vi "Create Hysteresis Results Summary Table.vi"(8 "error in (no error)":errorcluster, 11 "Hysteresis Results":T1[](array[typedef]) {"Hysteresis Percent FS" format="%#_3g"}) -> (0 "error out":errorcluster, 3 "Hysteresis Table":string[][](array[string]))   [LabVIEW 2026, in "Analysis.lvlib"]
uses:
  Analysis.lvlib
  Hysteresis Result.ctl
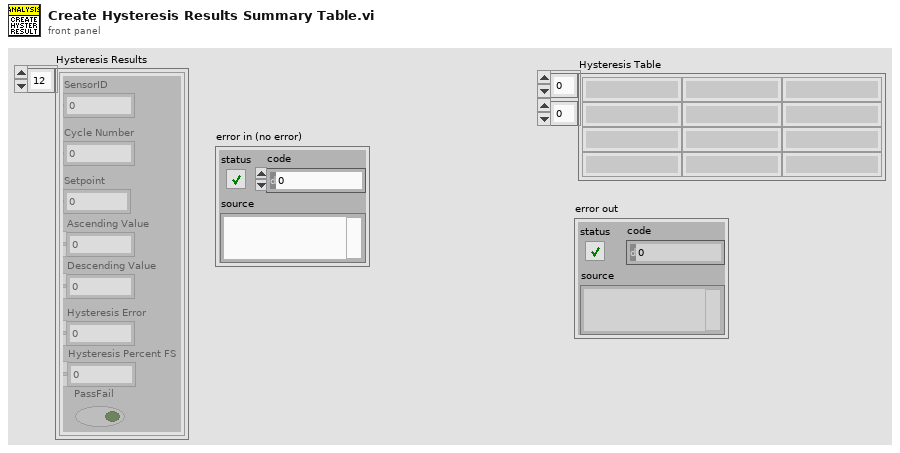
[diagram p1: front panel]
types:
  T1 = typedef "Analysis.lvlib/Hysteresis Result.ctl" = cluster{"Setpoint":dbl, "Ascending Value":dbl, "Cycle Number":i32, "SensorID":i32, "Descending Value":dbl, "Hysteresis Error":dbl, "Hysteresis Percent FS":dbl, "PassFail":bool}
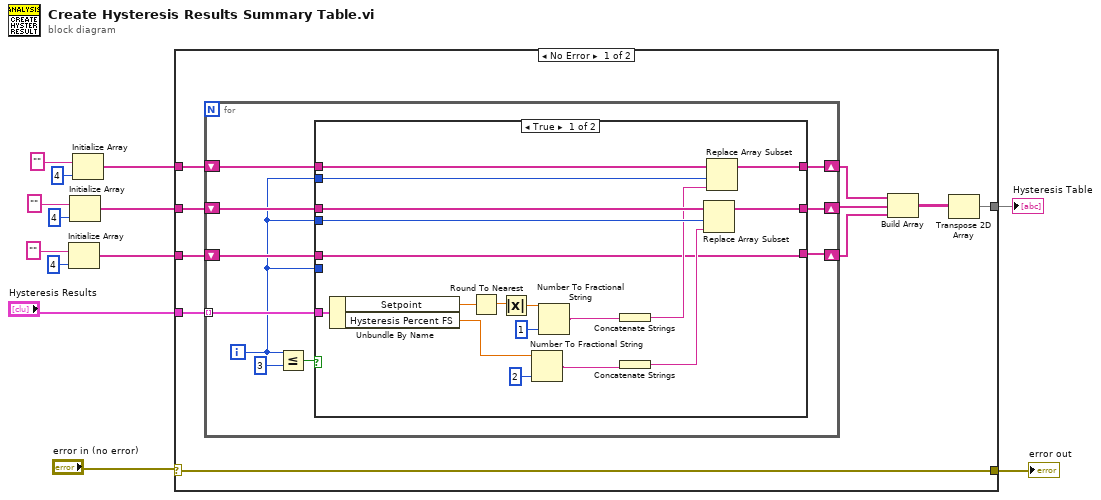
[diagram p0: block diagram]
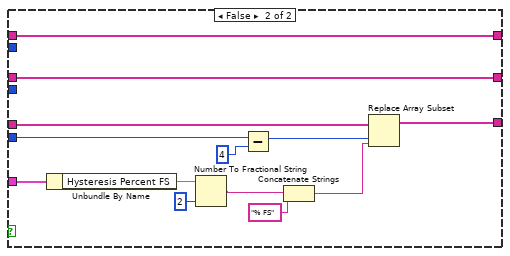
[diagram p2: hidden frame]
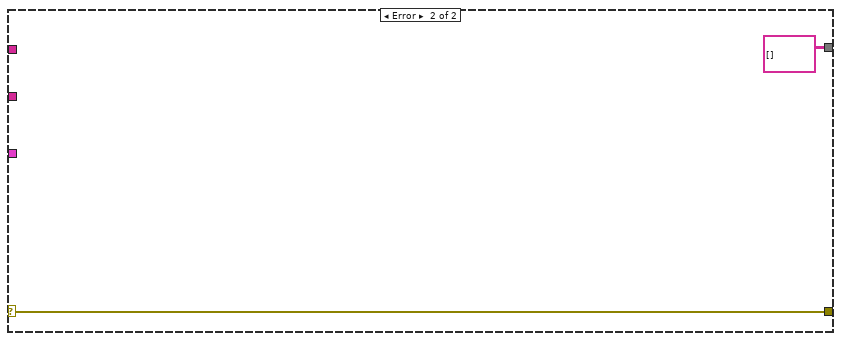
[diagram p3: hidden frame]
diagram:
  n1 = Initialize Array("" ("element"), 4 ("dimension size")) -> (w5:string[])
  n2 = Initialize Array("" ("element"), 4 ("dimension size")) -> (w8:string[])
  n3 = Initialize Array("" ("element"), 4 ("dimension size")) -> (w11:string[])
  n4 = case shown="No Error" "error in (no error)" {
    selector: "error in (no error)" -> [w14 w66]
    tunnel: w11 -> [w23 _]
    tunnel: w8 -> [w22 _]
    tunnel: w5 -> [w21 _]
    tunnel: "Hysteresis Results" -> [w17 _]
    tunnel: [w15 string[][] []] -> w3
    tunnel: [w14 w66] -> w1
    frame No Error {
      n5 = for {
        tunnel: w17 -> [w33] mode=indexing
        shift-right: [w27] -> w20
        shift-left: w23 -> [w30]
        shift-right: [w28] -> w19
        shift-left: w22 -> [w29]
        shift-right: [w24] -> w18
        shift-left: w21 -> [w26]
        i -> [w25]
        n6 = Less Or Equal?(x=w25, y=3) -> (x <= y?=w31:bool)
        n7 = case shown="True" w31 {
          tunnel: w33 -> [w51 w64]
          tunnel: w30 -> [w42 w59]
          tunnel: w29 -> [w47 w58]
          tunnel: w25 -> [w46 _]
          tunnel: [w45 w58] -> w28
          tunnel: [w41 w59] -> w27
          tunnel: w25 -> [w40 _]
          tunnel: w26 -> [w39 w57]
          tunnel: w25 -> [_ w54]
          tunnel: [w39 w55] -> w24
          frame True {
            n8 = Unbundle By Name(w51) -> ("Setpoint"=w37:dbl, "Hysteresis Percent FS"=w49:dbl)
            n9 = Round To Nearest(number=w37) -> (nearest integer value=w35:dbl)
            n10 = Absolute Value(x=w35) -> (abs(x)=w34:dbl)
            n11 = Number To Fractional String(number=w49, precision (6)=i16 2) -> (F-format string=w48:string)  [unwired: 2 in]
            n12 = Number To Fractional String(number=w34, precision (6)=i16 1) -> (F-format string=w50:string)  [unwired: 2 in]
            n13 = Concatenate Strings(w50) -> (w44:string)
            n14 = Concatenate Strings(w48) -> (w43:string)
            n15 = Replace Array Subset(array=w47, new element=w43, index=w46) -> (w45:string[])
            n16 = Replace Array Subset(array=w42, new element=w44, index=w40) -> (w41:string[])
          }
          frame False {
            n17 = Unbundle By Name(w64) -> ("Hysteresis Percent FS"=w63:dbl)
            n18 = Number To Fractional String(number=w63, precision (6)=i16 2) -> (F-format string=w60:string)  [unwired: 2 in]
            n19 = Subtract(x=w54, y=4 ("precision (6)")) -> (x-y=w52:i32)
            n20 = Concatenate Strings(w60, "% FS" ("element")) -> (w56:string)
            n21 = Replace Array Subset(array=w57, new element=w56, index=w52) -> (w55:string[])
          }
        }
      }
      n22 = Build Array(w20, w19, w18) -> (w16:string[][])
      n23 = Transpose 2D Array(2D array=w16) -> (transposed array=w15:string[][])
    }
    frame Error {
    }
  }
  "Hysteresis Table" <- w3
  "error out" <- w1
